vi "Mass Dispense Control (SubVI).vi"(0 "Weight (Grams)":dbl, 1 "Dispense Setpoint (%)":dbl=2.0, 2 "Fill Setpoint (g)":dbl=1000.0, 3 "Settings":T2={"ON Settings"={"Enable Dynamic Setpoint?"=TRUE, "Enable Dynamic Dispense Time?"=TRUE, "Enable Drain Rate Functions"=TRUE, "Dispense Sample Time (s)"=0.1, "Mass Average Samples"=20, "ON Timeout (sec)"=300.0, "1st Setpoint (% of Target)"=90.0, "2nd Setpoint (% of Target)"=95.0, "3rd Setpoint (% of Target)"=100.0, "Measure Dispense Delay (sec)"=10.0, "Minimum Spray Time (s)"=2.0, "Pump Reverse Time (s)"=10.0}, "OFF Settings"={"Drain Sample Time (s)"=0.1, "Drain Rate Ave Size"=100, "Drain Rate Limits (± g/sec)"=100.0, "Level Slope Range (± g/sec)"=0.05, "OFF Timeout (sec)"=300.0, "Near SP Slope Level (± g/sec)"=0.005, "Near Setpoint Threshold (%)"=99.0}, "Overshoot Settings"={"Time Limit (s)"=30.0, "Container MAX (g)"=1500.0, "Max FILL Slope (+/- g/sec)"=100.0, "% Overshot to Enable (>)"=3.0}, "FILL Timeout (s)"=300.0, "Full \nSettle Time (s)"=30.0, "Pre-Hydrate \nSpray Time (s)"=0.0, "Pre-Hydrate \nWait Time (s)"=10.0, "m Value "=1.0, "b Value"=0.0, "Enable Overshoot Adjust?"=FALSE} {"ON Settings"."Pump Reverse Time (s)" min=0.0 max=60.0; "OFF Settings"."Near SP Slope Level (± g/sec)" format="%.3g"; "OFF Settings"."Level Slope Range (± g/sec)" format="%.3g"}, 4 "Product Weight (g)":dbl, 6 "STOP Dispense":bool, 8 "START Dispense":bool) -> (11 "Spray Count":i32, 14 "Signals":T1={"Dispense"=FALSE, "Fill"=FALSE, "Spray"=FALSE, "Drain"=TRUE, "Complete"=FALSE, "Fill Error"=FALSE, "Disp. Error"=FALSE, "Fill Timeout"=FALSE, "Disp. Timeout"=FALSE, "Purge"=TRUE}, 16 "Values":T5 {"Drain Time (s)" format="%.2f"; "Drain Rate (g/sec)" format="%.2f"; "Time Elapsed (s)" format="%.2f"; "Time Target (s)" format="%.2f"; "Dynamic Setpoint (g)" format="%.2f"; "Static Setpoint (g)" format="%.2f"; "Grams to Setpoint" format="%.2f"; "Adjusted Mass (g)" format="%.2f"; "Dispense Rate (g/sec)" format="%.2f"; "Fill Mass (g)" format="%.2f"; "Fill Rate (g/sec)" format="%.2f"}, 17 "Product Values":T3, 18 "Hydration (g)":dbl, 19 "Dispense Mode":T4(ring))   [LabVIEW 2011]
panel:
  # "ONLY ADJUST\nBOLD VALUES!"
  # "Corrected Mass = SDC Mass * m + b"
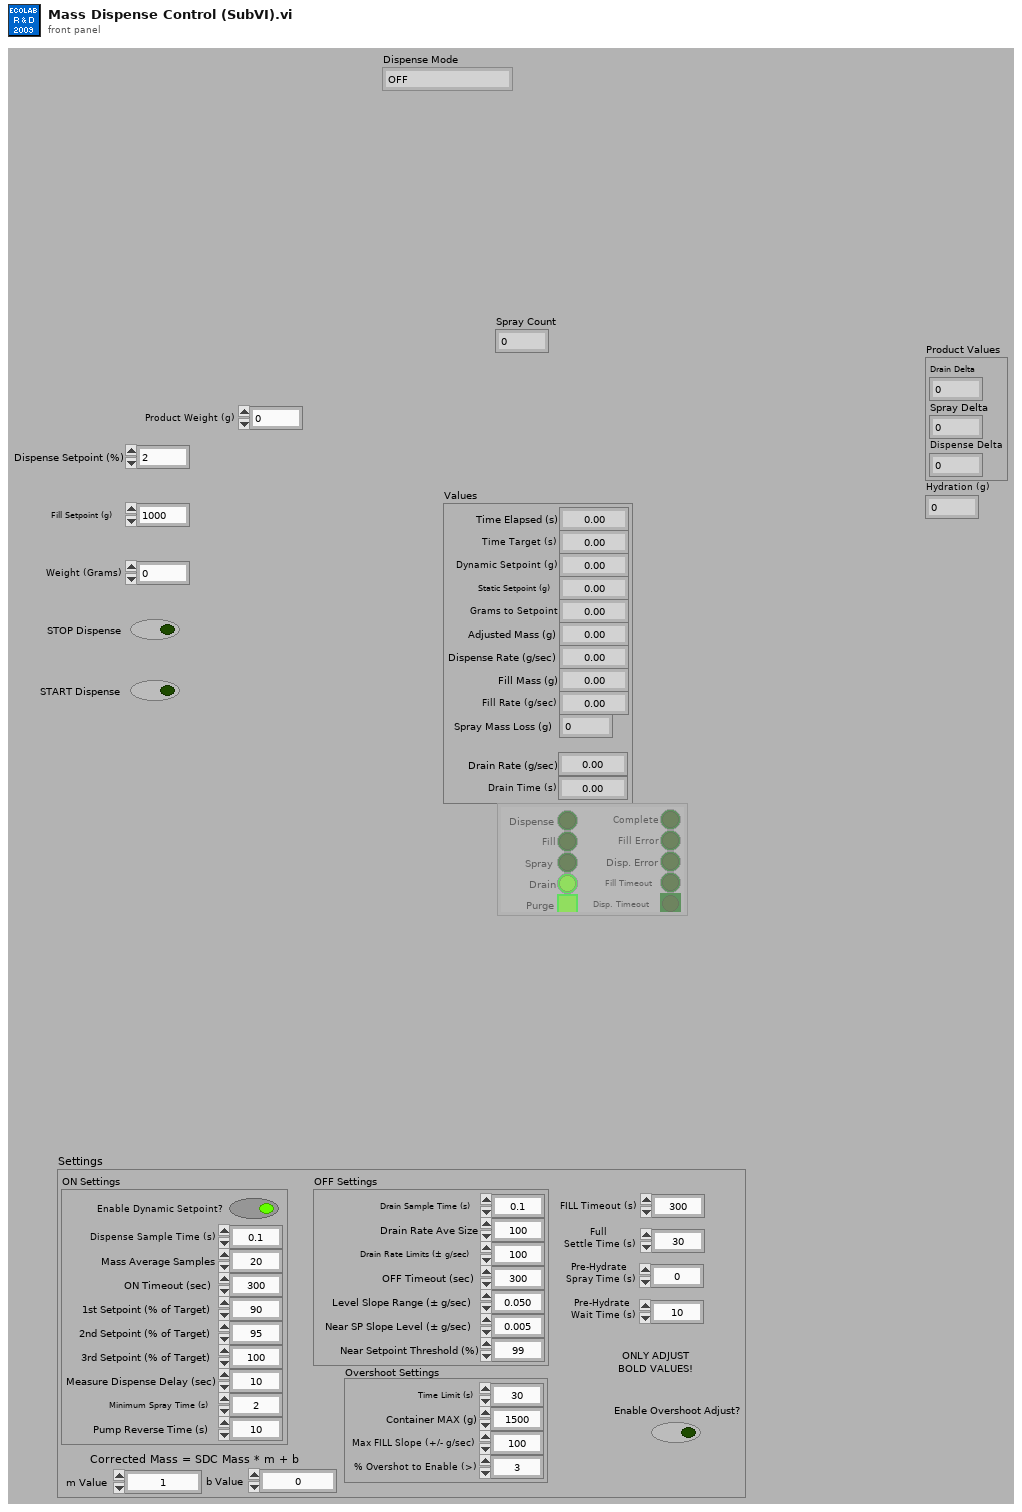
[diagram p1: front panel]
types:
  T1 = cluster{"Dispense":bool, "Fill":bool, "Spray":bool, "Drain":bool, "Complete":bool, "Fill Error":bool, "Disp. Error":bool, "Fill Timeout":bool, "Disp. Timeout":bool, "Purge":bool}
  T2 = cluster{"ON Settings":cluster{"Enable Dynamic Setpoint?":bool, "Enable Dynamic Dispense Time?":bool, "Enable Drain Rate Functions":bool, "Dispense Sample Time (s)":dbl, "Mass Average Samples":i32, "ON Timeout (sec)":dbl, "1st Setpoint (% of Target)":dbl, "2nd Setpoint (% of Target)":dbl, "3rd Setpoint (% of Target)":dbl, "Measure Dispense Delay (sec)":dbl, "Minimum Spray Time (s)":dbl, "Pump Reverse Time (s)":dbl}, "OFF Settings":cluster{"Drain Sample Time (s)":dbl, "Drain Rate Ave Size":i32, "Drain Rate Limits (± g/sec)":dbl, "Level Slope Range (± g/sec)":dbl, "OFF Timeout (sec)":dbl, "Near SP Slope Level (± g/sec)":dbl, "Near Setpoint Threshold (%)":dbl}, "Overshoot Settings":cluster{"Time Limit (s)":dbl, "Container MAX (g)":dbl, "Max FILL Slope (+/- g/sec)":dbl, "% Overshot to Enable (>)":dbl}, "FILL Timeout (s)":dbl, "Full \nSettle Time (s)":dbl, "Pre-Hydrate \nSpray Time (s)":dbl, "Pre-Hydrate \nWait Time (s)":dbl, "m Value ":dbl, "b Value":dbl, "Enable Overshoot Adjust?":bool}
  T3 = cluster{"Drain Delta":dbl, "Spray Delta":dbl, "Dispense Delta":dbl}
  T4 = enum16{"OFF", "INITIAL", "FILL", "DISPENSE", "ADJUST"}
  T5 = cluster{"Time Elapsed (s)":dbl, "Time Target (s)":dbl, "Dynamic Setpoint (g)":dbl, "Static Setpoint (g)":dbl, "Grams to Setpoint":dbl, "Adjusted Mass (g)":dbl, "Dispense Rate (g/sec)":dbl, "Fill Mass (g)":dbl, "Fill Rate (g/sec)":dbl, "Spray Mass Loss (g)":dbl, "Drain Rate (g/sec)":dbl, "Drain Time (s)":dbl}
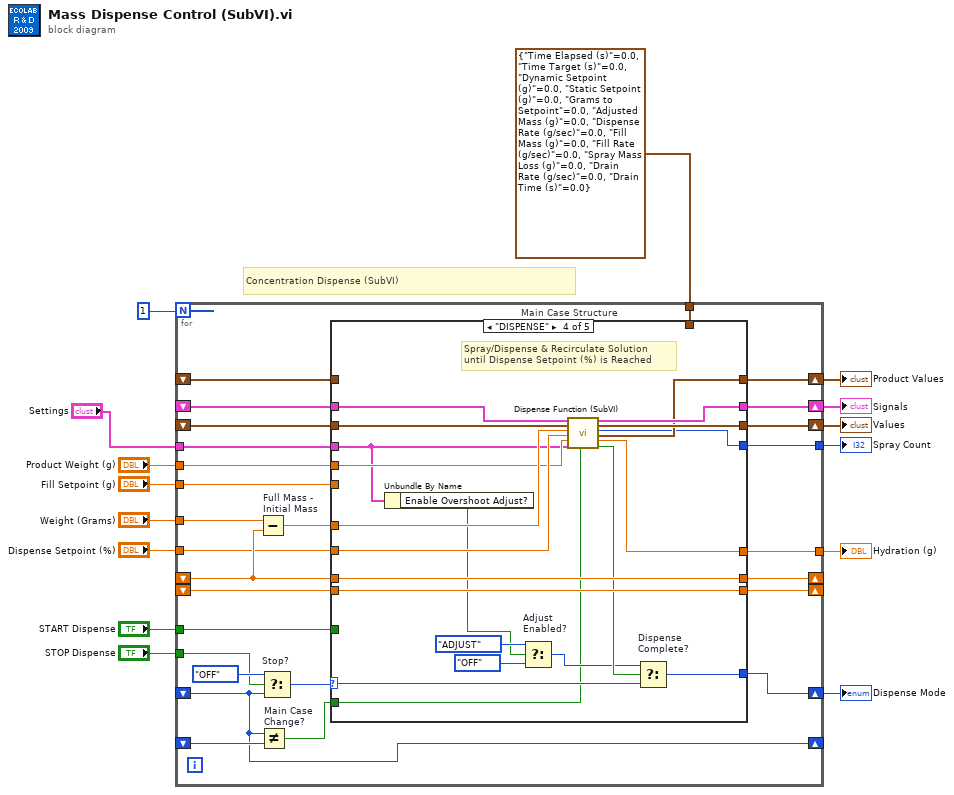
[diagram p0: block diagram]
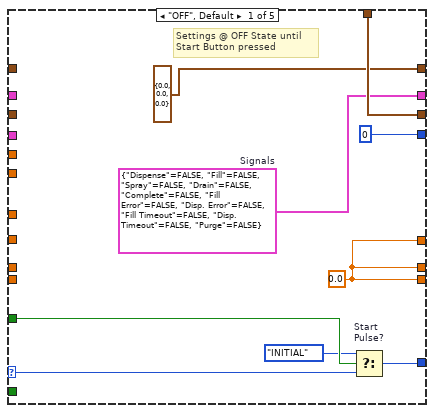
[diagram p2: hidden frame]
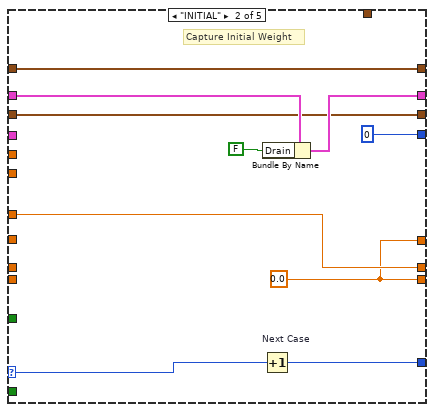
[diagram p3: hidden frame]
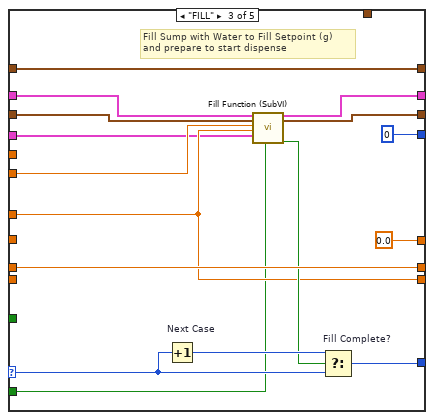
[diagram p4: hidden frame]
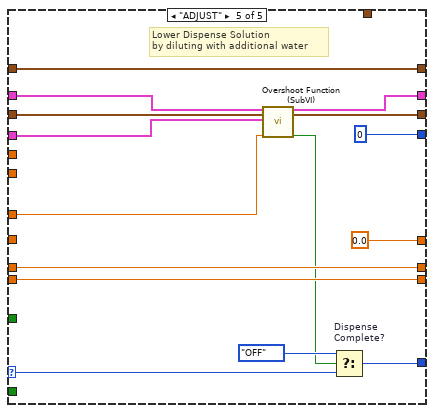
[diagram p5: hidden frame]
diagram:
  # "Concentration Dispense (SubVI)"
  n1 = for {
    N: 1 -> [_]
    tunnel: "Weight (Grams)" -> [w35]
    shift-right: [w42] -> w7
    shift-left: _ -> [w17]
    tunnel: "Fill Setpoint (g)" -> [w30]
    tunnel: "Dispense Setpoint (%)" -> [w26]
    shift-right: [w41] -> w1
    shift-left: _ -> [w31]
    shift-right: [w40] -> _
    shift-left: _ -> [w36]
    tunnel: "START Dispense" -> [w39]
    tunnel: "STOP Dispense" -> [w37]
    shift-right: [w34] -> _
    shift-left: _ -> [w33]
    tunnel: "Settings" -> [w25]
    tunnel: T5 {"Time Elapsed (s)"=0.0, "Time Target (s)"=0.0, "Dynamic Setpoint (g)"=0.0, "Static Setpoint (g)"=0.0, "Grams to Setpoint"=0.0, "Adjusted Mass (g)"=0.0, "Dispense Rate (g/sec)"=0.0, "Fill Mass (g)"=0.0, "Fill Rate (g/sec)"=0.0, "Spray Mass Loss (g)"=0.0, "Drain Rate (g/sec)"=0.0, "Drain Time (s)"=0.0} -> [w29]
    shift-right: [w28] -> w8
    shift-left: _ -> [w27]
    tunnel: "Product Weight (g)" -> [w24]
    shift-right: [w23] -> w5
    shift-left: _ -> [w22]
    tunnel: [w21] -> w4
    shift-right: [w17] -> _
    shift-left: _ -> [w20]
    tunnel: [w16] -> w3
    n2 = Subtract "Full Mass -\nInitial Mass"(x=w35, y=w36) -> (x-y=w32:dbl)
    n3 = Not Equal? "Main Case\nChange?"(x=w17, y=w20) -> (x != y?=w18:bool)
    n4 = Select "Stop?"(t=T4."OFF" ("Mode (Read)"), s=w37, f=w17) -> (s? t:f=w19:T4)
    n5 = case "Main Case Structure" shown="\"DISPENSE\"" w19 {
      selector: w19 -> [w50 w61 w76 w95 w104]
      tunnel: w32 -> [_ w60 w70 w89 w103]
      tunnel: [w49 w59 w75 w98 w106] -> w42
      tunnel: w30 -> [_ _ w73 _ _]
      tunnel: [w43 w57 w69 w93 w110] -> w41
      tunnel: w31 -> [_ w58 w72 w94 w111]
      tunnel: [w45 w60 w74 w97 w113] -> w40
      tunnel: w36 -> [_ _ w74 w97 w113]
      tunnel: w39 -> [w51 _ _ _ _]
      tunnel: [w45 w53 w70 w96 w112] -> w34
      tunnel: w33 -> [_ _ _ w96 w112]
      tunnel: w29 -> [w48 _ _ _ _]
      tunnel: [w48 w55 w67 w90 w108] -> w28
      tunnel: w27 -> [_ w55 w68 w92 w109]
      tunnel: w26 -> [_ _ _ w88 _]
      tunnel: w25 -> [_ _ w62 w79 w99]
      tunnel: w24 -> [_ _ _ w84 _]
      tunnel: [T3 {"Drain Delta"=0.0, "Spray Delta"=0.0, "Dispense Delta"=0.0} ("Product Values") w54 w66 w83 w102] -> w23
      tunnel: w22 -> [_ w54 w66 _ w102]
      tunnel: [w45 w53 0.0 ("Hydration (g)") w82 0.0 ("Hydration (g)")] -> w21
      tunnel: w18 -> [_ _ w64 w81 _]
      tunnel: [0 ("Spray Count") 0 ("Spray Count") 0 ("Spray Count") w80 0 ("Spray Count")] -> w16
      frame "OFF", Default {
        w43 = T1 {"Dispense"=FALSE, "Fill"=FALSE, "Spray"=FALSE, "Drain"=FALSE, "Complete"=FALSE, "Fill Error"=FALSE, "Disp. Error"=FALSE, "Fill Timeout"=FALSE, "Disp. Timeout"=FALSE, "Purge"=FALSE}  # Signals
        w45 = 0.0 ("Weight (Grams)")
        # "Settings @ OFF State until\nStart Button pressed"
        n6 = Select "Start\nPulse?"(t=T4."INITIAL" ("Mode (Read)"), s=w51, f=w50) -> (s? t:f=w49:T4)
      }
      frame "INITIAL" {
        w53 = 0.0 ("Weight (Grams)")
        # "Capture Initial Weight"
        n7 = Increment "Next Case"(x=w61) -> (x+1=w59:T4)
        n8 = Bundle By Name(cluster=w58, "Drain"=FALSE) -> (w57:T1)
      }
      frame "FILL" {
        # "Fill Sump with Water to Fill Setpoint (g)\nand prepare to start dispense"
        n9 = Increment "Next Case"(x=w76) -> (x+1=w77:T4)
        n10 = call "Fill Function (SubVI).vi"("Signals IN"=w72, "Values IN"=w68, "FILL Setpoint (g)"=w73, "Measured Mass (g)"=w70, "Settings"=w62, "Main Case Change?"=w64) -> ("Signals OUT"=w69:T1, "Values OUT"=w67:T5, "Fill FN Complete"=w71:bool)  [unwired: 1 in, 10 out]
        n11 = Select "Fill Complete?"(t=w77, s=w71, f=w76) -> (s? t:f=w75:T4)
      }
      frame "DISPENSE" {
        # "Spray/Dispense & Recirculate Solution\nuntil Dispense Setpoint (%) is Reached"
        n12 = Unbundle By Name(w79) -> ("Enable Overshoot Adjust?"=w78:bool)
        n13 = Select "Adjust\nEnabled?"(t=T4."ADJUST" ("Mode (Read)"), s=w78, f=T4."OFF" ("Mode (Read)")) -> (s? t:f=w85:T4)
        n14 = call "Dispense Function (SubVI).vi"("Signals IN"=w94, "Values IN"=w92, "Measured Mass (g)"=w89, "Main Concentration Setpoint (%)"=w88, "Product Weight (g)"=w84, "Settings"=w79, "Main Case Change?"=w81) -> ("Signals OUT"=w93:T1, "Values OUT"=w90:T5, "Spray Count"=w80:i32, "Product Values"=w83:T3, "Hydration (g)"=w82:dbl, "Dispense Complete?"=w91:bool)  [unwired: 7 out]
        n15 = Select "Dispense\nComplete?"(t=w85, s=w91, f=w95) -> (s? t:f=w98:T4)
      }
      frame "ADJUST" {
        # "Lower Dispense Solution\nby diluting with additional water"
        n16 = call "Overshoot Function (SubVI).vi"("Signals IN"=w111, "Values IN"=w109, "Settings"=w99, "Measured Mass (g)"=w103) -> ("Signals OUT"=w110:T1, "Values OUT"=w108:T5, "Complete"=w105:bool)  [unwired: 4 in, 9 out]
        n17 = Select "Dispense\nComplete?"(t=T4."OFF" ("Mode (Read)"), s=w105, f=w104) -> (s? t:f=w106:T4)
      }
    }
  }
  "Values" <- w8
  "Dispense Mode" <- w7
  "Product Values" <- w5
  "Hydration (g)" <- w4
  "Spray Count" <- w3
  "Signals" <- w1
